vi "ACQuire_COMPlete.vi"(7 "Write?":bool, 8 "Error":errorcluster caption="错误输入（无错误）", 11 "VISA resource name":refnum<visa-resource-name>) -> (0 "Error out":errorcluster, 2 "COMPlete out":u32, 3 "VISA resource name out":refnum<visa-resource-name>)   [LabVIEW 2020]
doc: "数据包数"
panel:
  out "读取缓冲区":string
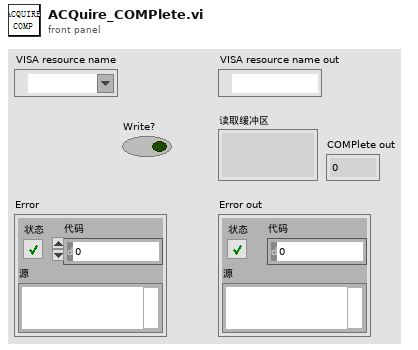
[diagram p1: front panel]
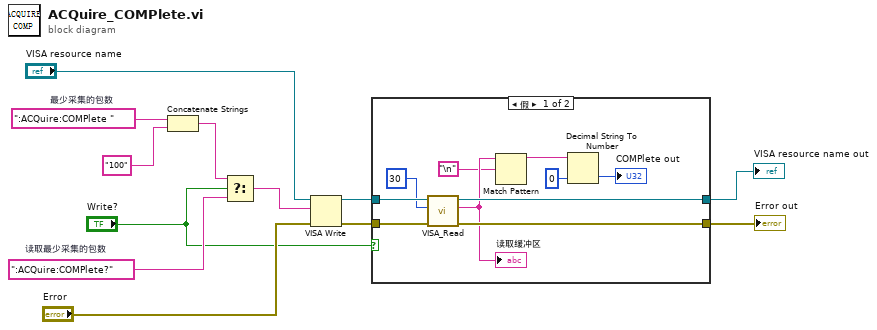
[diagram p0: block diagram]
diagram:
  w9 = ":ACQuire:COMPlete?"  # 读取最少采集的包数
  w11 = ":ACQuire:COMPlete "  # 最少采集的包数
  n1 = Concatenate Strings(w11, "100" ("字符串")) -> (w10:string)
  n2 = Select(t=w10, s="Write?", f=w9) -> (s? t:f=w8:string)
  n3 = VISA Write(VISA resource name="VISA resource name", write buffer=w8, error in (no error)="Error") -> (VISA resource name out=w4:refnum<visa-resource-name>, error out=w6:errorcluster)  [unwired: 1 out]
  n4 = case shown="假" "Write?" {
    tunnel: w4 -> [w22 w24]
    tunnel: w6 -> [w21 w23]
    tunnel: [w19 w23] -> w5
    tunnel: [w20 w24] -> w1
    frame False {
      n5 = call "VISA_Read.vi"("Error"=w21, "字节总数"=u32 30, "VISA resource name"=w22) -> ("Error out"=w19:errorcluster, "读取缓冲区"=w18:string, "VISA resource name out"=w20:refnum<visa-resource-name>)  [unwired: 6 in]
      "读取缓冲区" <- w18
      n6 = Match Pattern(string=w18, regular expression="\n") -> (before substring=w15:string)  [unwired: 1 in, 3 out]
      n7 = Decimal String To Number(string=w15, default (0L)=u32 0 ("默认(0 I32)")) -> (number=→"COMPlete out":u32)  [unwired: 1 in, 1 out]
    }
    frame True {
    }
  }
  "VISA resource name out" <- w1
  "Error out" <- w5
